vi "Teardown.vi"(11 "jettl Event Actor in":refnum<class "jettl Event Actor.lvclass">) -> (0 "error out":errorcluster)   [LabVIEW 2021, in "jettl Event Actor.lvclass"]
uses:
  jettl Event Actor.lvclass
  jettl Event Actor.lvclass/jettl Event Actor.ctl
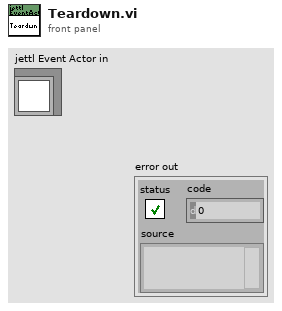
[diagram p1: front panel]
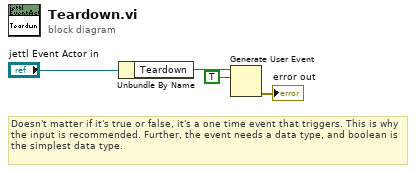
[diagram p0: block diagram]
diagram:
  # "Doesn't matter if it's true or false, it's a one time event that triggers. This is why the input is recommended. Further, the event needs a data type, and boolean is the simplest data type."
  n1 = Unbundle By Name("jettl Event Actor in") -> ("Teardown"=w2:refnum<user-event>)
  n2 = Generate User Event(user event=w2, event data cluster=TRUE ("event data")) -> (error out=→"error out":errorcluster)  [unwired: 2 in, 1 out]
